vi "XY graph cursor_0209.vi"() -> ()   [LabVIEW 2021]
uses:
  <vilib>/Utility/miscctls.llb/LVCursorListTypeDef.ctl
panel:
  in  "Plot1 Y-Offset":dbl
  in  "Plot1  X-Offset":dbl
  in  "Plot1 Style":u8=4
  in  "Plot1 Point Style":u8=13
  in  "Plot 0  Y-Offset":dbl
  in  "Plot 0 X-Offset":dbl
  in  "Plot 0 Style":u8
  in  "Plot 0 Point Style":u8
  in  "Cursor List":T1=[{"Name"="", "Color"=0, "Style"=0, "Point Style"=0, "Name Visible"=TRUE, "Allow Drag"=FALSE, "Cursor Mode"=0, "Plot"=0, "Index"=0, "Position"={"X"=0.0, "Y"=0.0}, "X Scale"=0, "Y Scale"=0, "Watch Plots"=[], "Watch All Plots"=FALSE, "Plot Area"=0, "Label Offset"={"X"=8.0, "Y"=0.05}}]
  out "XY Graph":cluster{i32[], dbl[]}[](graph)
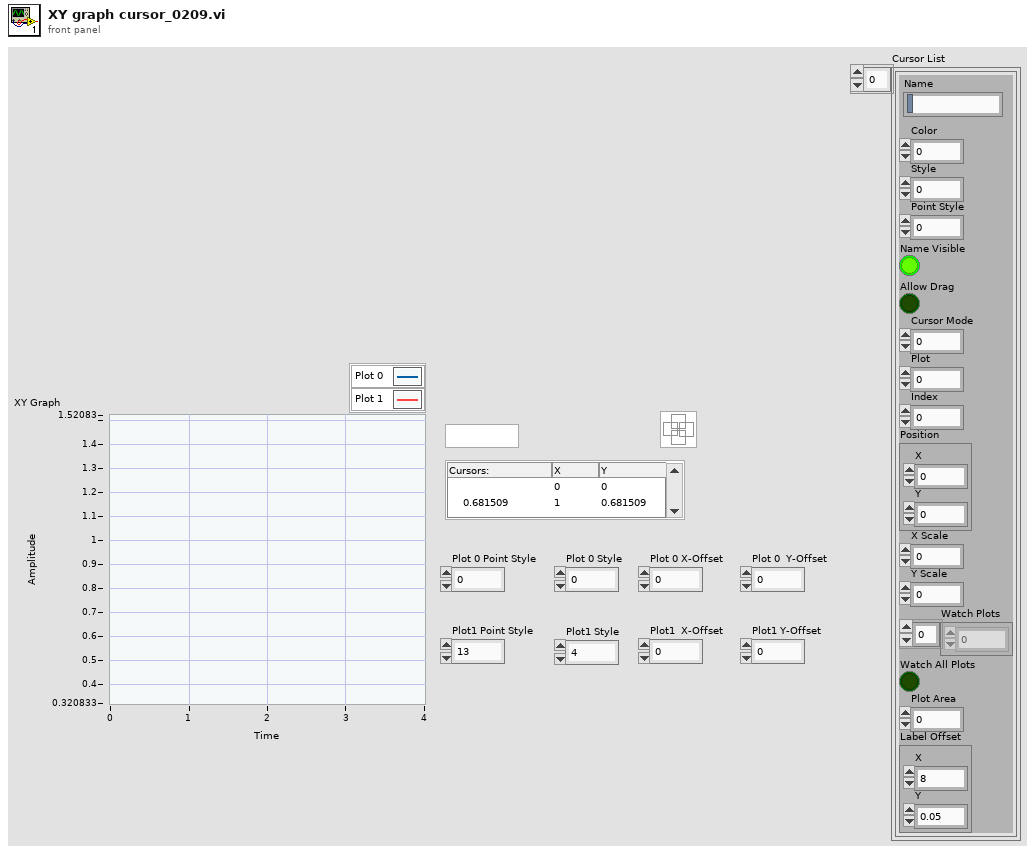
[diagram p1: front panel]
types:
  T1 = typedef "LVCursorListTypeDef.ctl" = cluster{"Name":string, "Color":u32, "Style":u8, "Point Style":u8, "Name Visible":bool, "Allow Drag":bool, "Cursor Mode":u32, "Plot":i32, "Index":i32, "Position":cluster{"X":dbl, "Y":dbl}, "X Scale":u32, "Y Scale":u32, "Watch Plots":i32[], "Watch All Plots":bool, "Plot Area":i32, "Label Offset":cluster{"X":dbl, "Y":dbl}}[]
  T2 = cluster{"Name":string, "Color":u32, "Style":u8, "Point Style":u8, "Name Visible":bool, "Allow Drag":bool, "Cursor Mode":u32, "Plot":i32, "Index":i32, "Position":cluster{"X":dbl, "Y":dbl}, "X Scale":u32, "Y Scale":u32, "Watch Plots":i32[], "Watch All Plots":bool, "Plot Area":i32, "Label Offset":cluster{"X":dbl, "Y":dbl}}
  T3 = cluster{"Name":string, "Color":u32, "Style":u8, "Point Style":u8, "Name Visible":bool, "Allow Drag":bool, "Cursor Mode":u32, "Plot":i32, "Index":i32, "Position":cluster{"X":dbl, "Y":dbl}, "X Scale":u32, "Y Scale":u32, "Watch Plots":i32[], "Watch All Plots":bool, "Plot Area":i32, "Label Offset":cluster{"X":dbl, "Y":dbl}}[]
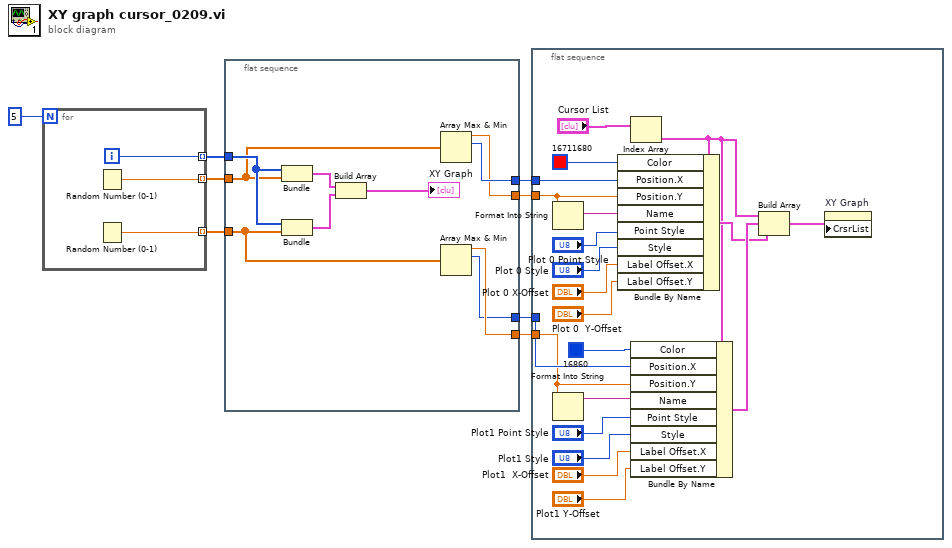
[diagram p0: block diagram]
diagram:
  n1 = for {
    N: 5 -> [_]
    tunnel: [w11] -> w4 mode=indexing
    tunnel: [w10] -> w3 mode=indexing
    tunnel: [w9] -> w5 mode=indexing
    i -> [w9]
    n2 = Random Number (0-1)() -> (number: 0 to 1=w11:dbl)
    n3 = Random Number (0-1)() -> (number: 0 to 1=w10:dbl)
  }
  n4 = flat-sequence {
    tunnel: [w21] -> w7
    tunnel: [w20] -> w6
    tunnel: w5 -> [w18]
    tunnel: w4 -> [w15]
    tunnel: w3 -> [w14]
    tunnel: [w13] -> w2
    tunnel: [w12] -> w1
    frame #0 {
      n5 = Bundle(w18, w15) -> (w19:cluster{i32[], dbl[]})  [unwired: 1 in]
      n6 = Bundle(w18, w14) -> (w17:cluster{i32[], dbl[]})  [unwired: 1 in]
      n7 = Build Array(w19, w17) -> (→"XY Graph":cluster{i32[], dbl[]}[])
      n8 = Array Max & Min(array=w15) -> (max value=w20:dbl, max index (indices)=w21:i32)  [unwired: 2 out]
      n9 = Array Max & Min(array=w14) -> (max value=w13:dbl, max index (indices)=w12:i32)  [unwired: 2 out]
    }
  }
  n10 = flat-sequence {
    tunnel: w7 -> [w41]
    tunnel: w6 -> [w39]
    tunnel: w2 -> [w33]
    tunnel: w1 -> [w34]
    frame #0 {
      n11 = Format Into String(w39) -> (resulting string=w40:string)  [unwired: 3 in, 1 out]
      n12 = Format Into String(w33) -> (resulting string=w36:string)  [unwired: 3 in, 1 out]
      n13 = Index Array(array="Cursor List") -> (element=w22:T2)  [unwired: 1 in]
      n14 = Bundle By Name(cluster=w22, "Color"=u32 16711680, "Position.X"=w41, "Position.Y"=w39, "Name"=w40, "Point Style"="Plot 0 Point Style", "Style"="Plot 0 Style", "Label Offset.X"="Plot 0 X-Offset", "Label Offset.Y"="Plot 0  Y-Offset") -> (w24:T2)
      n15 = Bundle By Name(cluster=w22, "Color"=u32 16860, "Position.X"=w34, "Position.Y"=w33, "Name"=w36, "Point Style"="Plot1 Point Style", "Style"="Plot1 Style", "Label Offset.X"="Plot1  X-Offset", "Label Offset.Y"="Plot1 Y-Offset") -> (w25:T2)
      n16 = Build Array(w22, w25, w24) -> (w26:T3)
      n17 = property on="XY Graph" class="XYGraph (strict)"("CrsrList"=w26) -> ()  [unwired: 2 in, 2 out]
    }
  }
